vi "GetEventList.vi"(7 "LabVIEW Web Service Request":refnum<class "Web Request.lvclass">, 8 "FID_2":string="5cf73d1ba0991c03a125caf0", 9 "FID_1":string="5cf73d1ba0991c03a125caef", 10 "SensorID":string="5cf73d1ba0991c03a125caee", 11 "AssetID":string="5cf73cf3a0991c03a125caeb") -> (3 "output":T1(array[cluster]))   [LabVIEW 2017]
uses:
  <vilib>/wsapi/Web Request.lvclass
  typedefs/Q_Message.ctl
  typedefs/Input IDs.ctl
panel:
  # "Use the Web Service Request input terminal to call the VIs on the Web Services palette. Do not remove it from the connector pane unless you don't need access to the palette."
  # "Each additional control wired to the connector pane will be available as an input in the URL. To include an indicator in terminal-mode output (the default setting), it must also be wired to the connector pane."
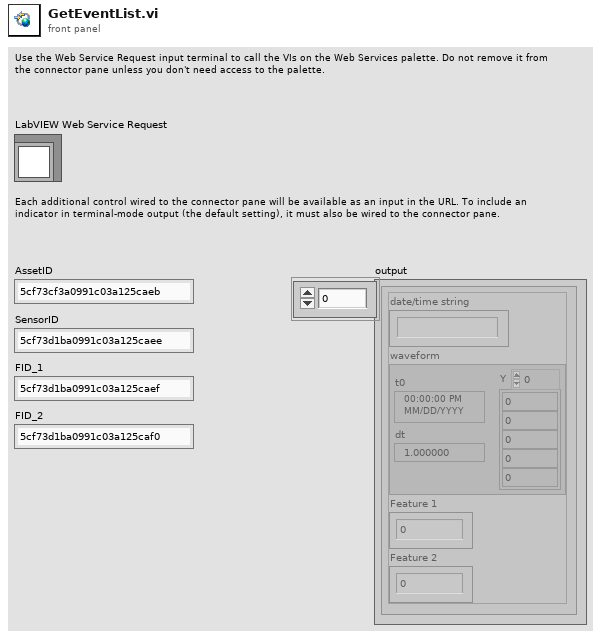
[diagram p1: front panel]
types:
  T1 = cluster{"date/time string":string, "waveform":waveform(sgl), "Feature 1":dbl, "Feature 2":dbl}[]
  T2 = typedef "Input IDs.ctl" = cluster{"Asset ID":string, "Sensor ID":string, "Feature id 1":string, "Feature id 2":string}
  T3 = typedef "Q_Message.ctl" = cluster{"Command":string, "Parameters":variant}
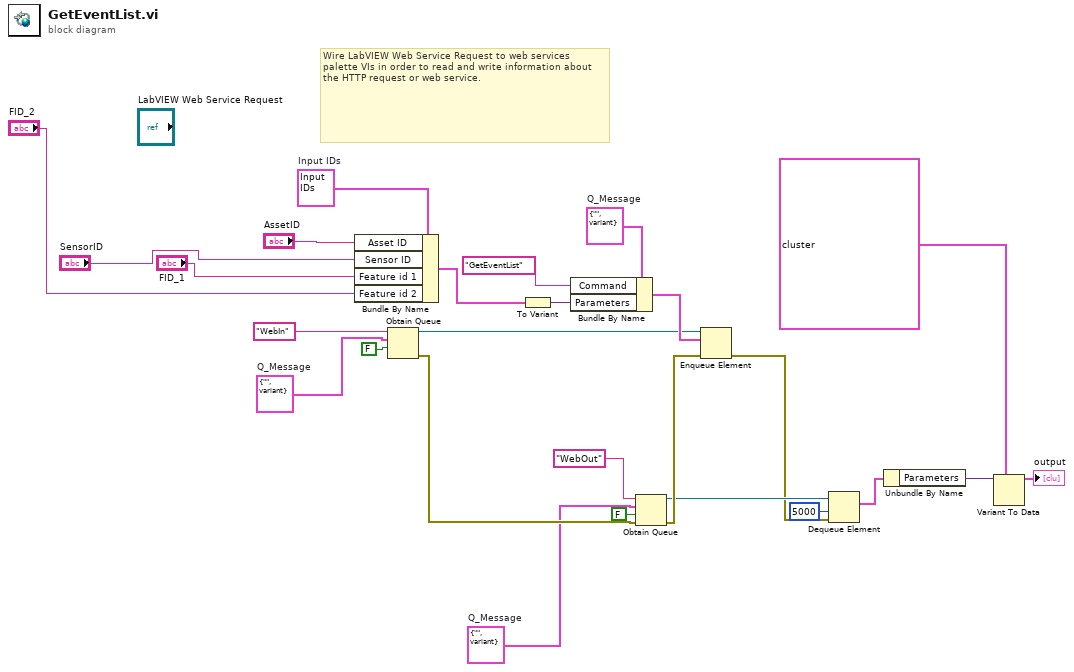
[diagram p0: block diagram]
diagram:
  w8 = T2 {"Asset ID"="5cf73cf3a0991c03a125caeb", "Sensor ID"="5cf73d1ba0991c03a125caee", "Feature id 1"="5cf73d1ba0991c03a125caef", "Feature id 2"="5cf73d1ba0991c03a125caf0"}  # Input IDs
  w11 = T3 {"Command"="", "Parameters"=variant}  # Q_Message
  w12 = T3 {"Command"="", "Parameters"=variant}  # Q_Message
  w13 = T3 {"Command"="", "Parameters"=variant}  # Q_Message
  # "Wire LabVIEW Web Service Request to web services palette VIs in order to read and write information about the HTTP request or web service."
  n1 = Bundle By Name(cluster=w8, "Asset ID"="AssetID", "Sensor ID"="SensorID", "Feature id 1"="FID_1", "Feature id 2"="FID_2") -> (w3:T2)
  n2 = Obtain Queue(name (unnamed)="WebIn", element data type=w13, create if not found? (T)=FALSE) -> (queue out=w21:refnum<queue>, error out=w19:errorcluster)  [unwired: 2 in, 1 out]
  n3 = To Variant(anything=w3) -> (Variant=w24:variant)
  n4 = Bundle By Name(cluster=w12, "Command"="GetEventList", "Parameters"=w24) -> (w23:T3)
  n5 = Obtain Queue(name (unnamed)="WebOut", element data type=w11, create if not found? (T)=FALSE, error in (no error)=w19) -> (queue out=w16:refnum<queue>, error out=w17:errorcluster)  [unwired: 1 in, 1 out]
  n6 = Enqueue Element(queue=w21, element=w23, error in (no error)=w17) -> (error out=w15:errorcluster)  [unwired: 1 in, 2 out]
  n7 = Dequeue Element(queue=w16, timeout in ms (-1)=5000, error in (no error)=w15) -> (element=w10:T3)  [unwired: 3 out]
  n8 = Unbundle By Name(w10) -> ("Parameters"=w9:variant)
  n9 = Variant To Data(type=T1 [{"date/time string"="10/7/2019 11:19:21 AM", "waveform"={"t0"=timestamp(3653263161 s since 1904-01-01), "dt"=0.000244140625, "Y"=array[245760 elements]}, "Feature 1"=5.12103817220665, "Feature 2"=0.0018771609136779158}, {"date/time string"="10/7/2019 12:09:59 PM", "waveform"={"t0"=timestamp(3653266199 s since 1904-01-01), "dt"=0.000244140625, "Y"=array[245760 elements]}, "Feature 1"=5.156669895439542, "Feature 2"=0.0018826798587614586}, {"date/time string"="10/7/2019 12:19:59 PM", "waveform"={"t0"=timestamp(3653266799 s since 1904-01-01), "dt"=0.000244140625, "Y"=array[245760 elements]}, "Feature 1"=4.736805719680169, "Feature 2"=0.0018771413916787638}, {"date/time string"="10/7/2019 12:24:59 PM", "waveform"={"t0"=timestamp(3653267099 s since 1904-01-01), "dt"=0.000244140625, "Y"=array[245760 elements]}, "Feature 1"=5.219101372687815, "Feature 2"=0.0018758608022062296}, {"date/time string"="10/7/2019 12:34:59 PM", "waveform"={"t0"=timestamp(3653267699 s since 1904-01-01), "dt"=0.000244140625, "Y"=array[245760 elements]}, "Feature 1"=5.2689887851738195, "Feature 2"=0.0018778648123666678}, {"date/time string"="10/7/2019 12:39:59 PM", "waveform"={"t0"=timestamp(3653267999 s since 1904-01-01), "dt"=0.000244140625, "Y"=array[245760 elements]}, "Feature 1"=4.749049177800525, "Feature 2"=0.0018708454227732057}, {"date/time string"="10/7/2019 12:44:59 PM", "waveform"={"t0"=timestamp(3653268299 s since 1904-01-01), "dt"=0.000244140625, "Y"=array[245760 elements]}, "Feature 1"=4.6568988407816265, "Feature 2"=0.0018792979598656902}] ("Output 2"), Variant=w9) -> (data=→"output":T1)  [unwired: 1 in, 1 out]
